vi "updateCounterRec.vi"(8 "error in (no error)":errorcluster, 10 "reset":bool, 11 "Logger in":refnum<class "Logger.lvclass">) -> (0 "error out":errorcluster, 3 "Logger out":refnum<class "Logger.lvclass">)   [LabVIEW 2018, in "Logger.lvclass"]
doc: "Update the counter of record. If the reset is True, the counter will be reset to 0. Otherwise, the counter will be added by 1."
uses:
  Logger.lvclass
  Logger.lvclass/Logger.ctl
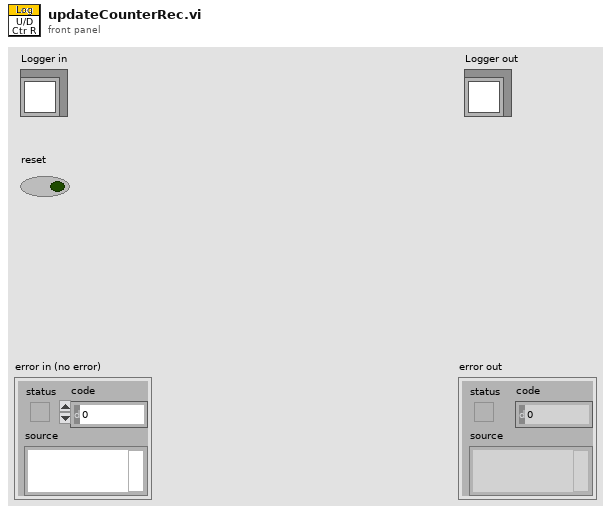
[diagram p1: front panel]
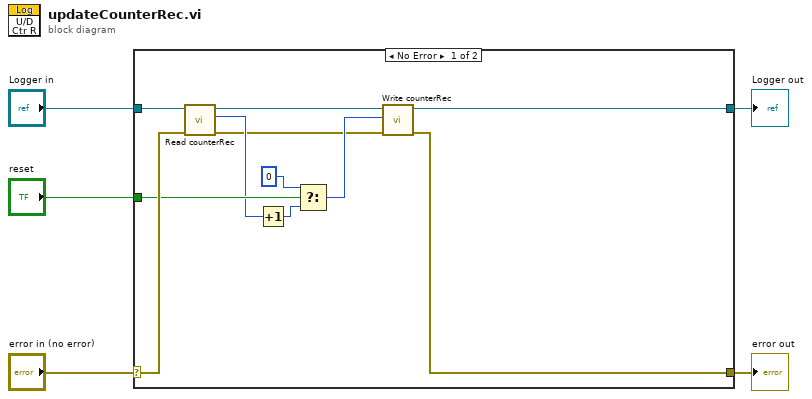
[diagram p0: block diagram]
diagram:
  n1 = case shown="No Error" "error in (no error)" {
    selector: "error in (no error)" -> [w15 w18]
    tunnel: [w7 w18] -> w4
    tunnel: [w6 w17] -> w2
    tunnel: "Logger in" -> [w16 w17]
    tunnel: "reset" -> [w14 _]
    frame No Error {
      n2 = call "Read counterRec.vi"("error in (no error)"=w15, "Logger in"=w16) -> ("error out"=w8:errorcluster, "counterRec"=w12:u32, "Logger out"=w10:refnum<class "Logger.lvclass">)  [unwired: 7 in]
      n3 = Increment(x=w12) -> (x+1=w13:u32)
      n4 = Select(t=u32 0, s=w14, f=w13) -> (s? t:f=w9:u32)
      n5 = call "Write counterRec.vi"("error in (no error)"=w8, "counterRec"=w9, "Logger in"=w10) -> ("error out"=w7:errorcluster, "Logger out"=w6:refnum<class "Logger.lvclass">)  [unwired: 7 in]
    }
    frame Error {
    }
  }
  "error out" <- w4
  "Logger out" <- w2
